vi "Lockin Engine.vi"(4 "order":i32=2, 6 "TC (s)":dbl=0.5, 9 "sampling info":cluster{"Fs":dbl, "#s":dbl}, 10 "Reference In":waveform(dbl)[](array[waveform]), 11 "Signal in":waveform(dbl)[](array[waveform])) -> (0 "filter fC (Hz)":dbl=0.3183098861837907, 3 "Results (X,Y,R,Theta)":dbl[][](array[numeric]))   [LabVIEW 2013]
uses:
  <vilib>/Analysis/baseanly.llb/Mean (DBL).vi
  <vilib>/Analysis/NI_AALBase.lvlib
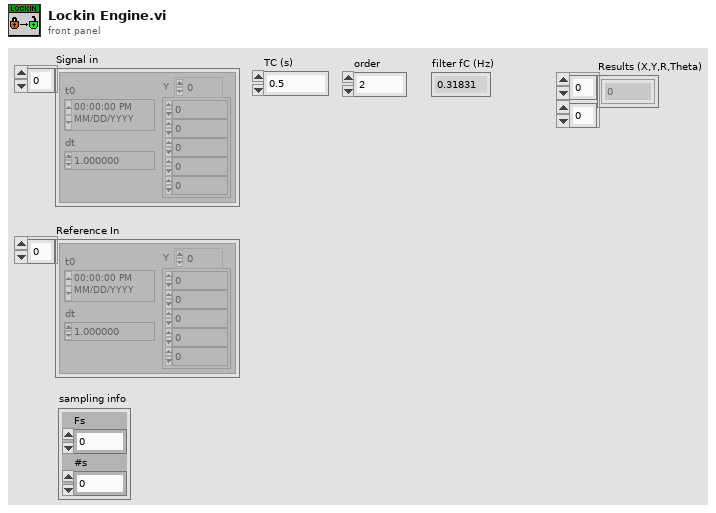
[diagram p1: front panel]
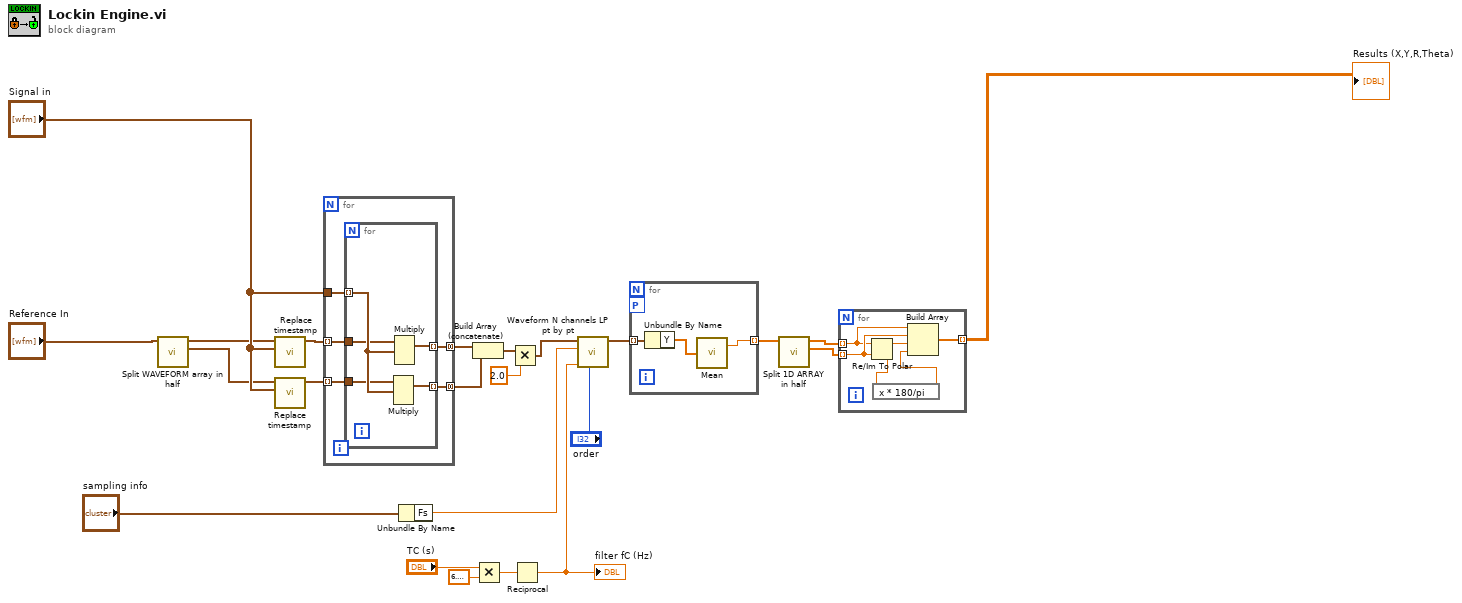
[diagram p0: block diagram]
diagram:
  n1 = call "Split WAVEFORM array in half.vi"("AO Array"="Reference In") -> ("Array"=w11:waveform(dbl)[], "Array 2"=w10:waveform(dbl)[])  [unwired: 9 in]
  n2 = call "Replace timestamp.vi"("Array in"="Signal in", "Array 2"=w10) -> ("Array"=w13:waveform(dbl)[])  [unwired: 9 in]
  n3 = call "Replace timestamp.vi"("Array in"="Signal in", "Array 2"=w11) -> ("Array"=w12:waveform(dbl)[])  [unwired: 9 in]
  n4 = for {
    tunnel: [w28] -> w6 mode=concatenating
    tunnel: [w27] -> w7 mode=concatenating
    tunnel: w12 -> [w26] mode=indexing
    tunnel: w13 -> [w25] mode=indexing
    tunnel: "Signal in" -> [w24]
    n5 = for {
      tunnel: [w33] -> w27 mode=indexing
      tunnel: w26 -> [w29]
      tunnel: w24 -> [w31] mode=indexing
      tunnel: w25 -> [w30]
      tunnel: [w32] -> w28 mode=indexing
      n6 = Multiply(1:w31, 2:w29) -> (0:w33:waveform(dbl))  [unwired: 1 in, 1 out]
      n7 = Multiply(1:w31, 2:w30) -> (0:w32:waveform(dbl))  [unwired: 1 in, 1 out]
    }
  }
  n8 = Unbundle By Name("sampling info") -> ("Fs"=w21:dbl)
  n9 = Build Array (concatenate)(w6, w7) -> (w8:waveform(dbl)[])
  n10 = Multiply(x="TC (s)", y=6.283185307179586) -> (x*y=w4:dbl)
  n11 = Multiply(x=w8, y=2.0) -> (x*y=w23:waveform(dbl)[])
  n12 = Reciprocal(x=w4) -> (1/x=w15:dbl)
  "filter fC (Hz)" <- w15
  n13 = call "Waveform N channels LP pt by pt.vi"("order"="order", "fl"=w15, "fs"=w21, "Array in"=w23) -> ("Array out"=w16:waveform(dbl)[])  [unwired: 7 in]
  n14 = for {
    tunnel: [w35] -> w17 mode=indexing
    workers-P: _ -> [_]
    tunnel: w16 -> [w34] mode=indexing
    n15 = Unbundle By Name(w34) -> ("Y"=w36:dbl[])
    n16 = call-poly <vilib>:"Mean.vi"("X"=w36) -> ("mean"=w35:dbl)  [unwired: 1 out]
  }
  n17 = call "Split 1D ARRAY in half.vi"("Array in"=w17) -> ("Array out"=w2:dbl[], "Array 3"=w1:dbl[])  [unwired: 9 in]
  n18 = for {
    tunnel: w1 -> [w39] mode=indexing
    tunnel: w2 -> [w41] mode=indexing
    tunnel: [w40] -> w9 mode=indexing
    n19 = Re/Im To Polar(2:w41, 3:w39) -> (0:w38:dbl, 1:w42:dbl)
    n20 = expression code="x * 180/pi"(w38) -> (w37:dbl)
    n21 = Build Array(w39, w41, w42, w37) -> (w40:dbl[])
  }
  "Results (X,Y,R,Theta)" <- w9
